vi "LDA+_An_Analysis_mode.vi"(6 "Second Graph":T2={"Plot 1"=1, "Plot 2"=2, "Save graph"=0, "Plot Type"=enum."Voltage trace"} {"Save graph" items=["Do not save plot", "Save plot"]; "Plot 2" items=["Nothing", "Prop 2 (U)"]; "Plot 1" items=["Nothing", "Prop 2 (U)"]}, 9 "First Graph":T2={"Plot 1"=1, "Plot 2"=2, "Save graph"=0, "Plot Type"=enum."Voltage trace"} {"Save graph" items=["Do not save plot", "Save plot"]; "Plot 2" items=["Nothing", "Prop 2 (U)"]; "Plot 1" items=["Nothing", "Prop 2 (U)"]}) -> (0 "Second Graph out":T2={"Plot 1"=1, "Plot 2"=2, "Save graph"=0, "Plot Type"=enum."Voltage trace"} {"Save graph" items=["Do not save plot", "Save plot"]; "Plot 2" items=["Nothing", "Prop 2 (U)"]; "Plot 1" items=["Nothing", "Prop 2 (U)"]}, 3 "First Graph out":T2={"Plot 1"=1, "Plot 2"=2, "Save graph"=0, "Plot Type"=enum."Voltage trace"} {"Save graph" items=["Do not save plot", "Save plot"]; "Plot 2" items=["Nothing", "Prop 2 (U)"]; "Plot 1" items=["Nothing", "Prop 2 (U)"]})   [LabVIEW 2010]
uses:
  Controls/Graph_Type.ctl
  Globals/Meas_global.vi
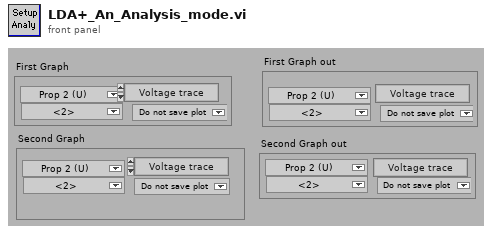
[diagram p1: front panel]
types:
  T1 = typedef "Graph_Type.ctl" = enum16{"Show no graph", "Voltage trace", "Velocity trace", "Vel histogram", "Spectrum", "f.E(f) v Log f", "Auto-Corr"}
  T2 = cluster{"Plot 1":u16, "Plot 2":u16, "Save graph":u16, "Plot Type":T1}
  T3 = typedef "Analysis_info_cluster.ctl" = cluster{"Colour":u32, "Inst type":T4, "Inst name":string, "Symbol":string, "Code name":string, "Extra Info":string, "Inst Array":T5, "Index":i32, "Voltage Index":i32, "Extra Titles":string[], "Extra Values":string[]}
  T4 = typedef "Inst_type.ctl" = enum16{"Propeller anemometer", "Raw voltage", "Pressure Transducer", "Pitot-static tube", "Preston tube", "Hot wire", "Cross wire 1", "Cross wire 2", "Generic Linear", "Generic Polynomial", "Generic BackPoly", "Fast FID", "Thermocouple", "Cold wire", "Pulsed Wire", "LDA Vel", "LDA Tran time", "LDA Arr time"}
  T5 = typedef "Instrument_Array.ctl" = enum16{"PWA", "LDA", "Analogue"}
  T6 = enum16{"Show no graph", "Voltage trace", "Velocity trace", " Vel histogram", "Spectrum", "f.E(f) v Log f", "Auto-Corr"}
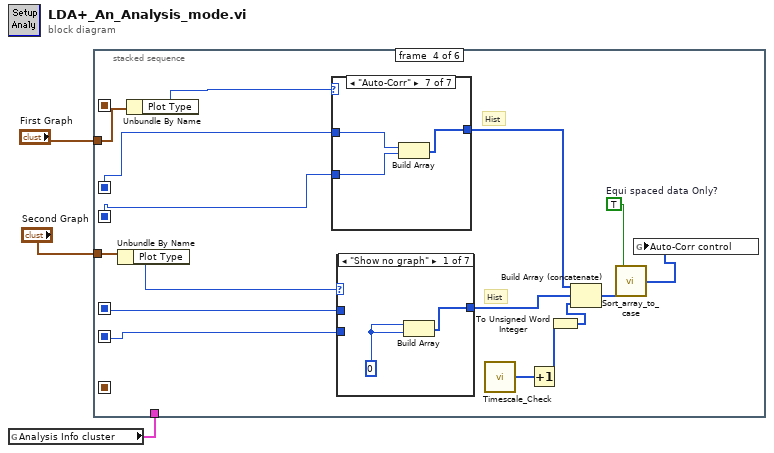
[diagram p0: block diagram]
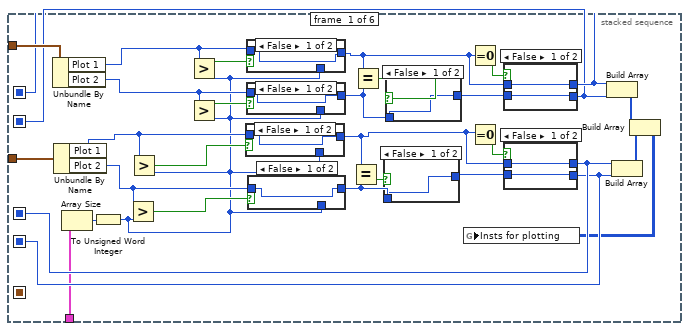
[diagram p2: hidden frame]
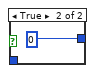
[diagram p5: hidden frame]
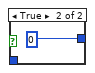
[diagram p10: hidden frame]
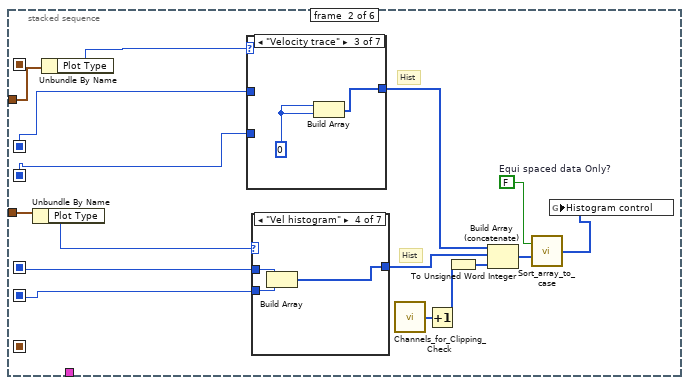
[diagram p11: hidden frame]
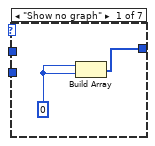
[diagram p12: hidden frame]
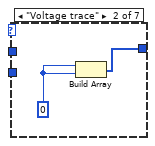
[diagram p13: hidden frame]
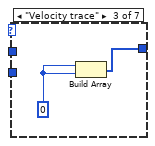
[diagram p14: hidden frame]
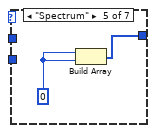
[diagram p15: hidden frame]
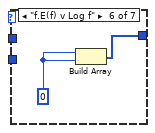
[diagram p16: hidden frame]
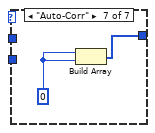
[diagram p17: hidden frame]
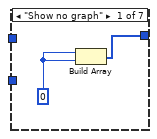
[diagram p18: hidden frame]
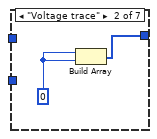
[diagram p19: hidden frame]
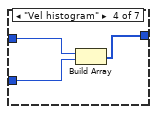
[diagram p20: hidden frame]
diagram:
  n1 = global read "Meas_global.vi" "Analysis Info cluster"() -> (w1:T3[])
  n2 = stacked-sequence {
    seq-local: [w15 _ _ _ _ _] -> [_ w64 w107 w155 w201 _]
    seq-local: [w14 _ _ _ _ _] -> [_ w63 w106 w154 w200 _]
    seq-local: [w10 _ _ _ _ _] -> [_ w66 w109 w157 w195 _]
    seq-local: [w9 _ _ _ _ _] -> [_ w65 w108 w156 w194 _]
    seq-local: [_ _ _ _ w191 _] -> [_ _ _ _ _ w229]
    seq-local: [_ _ _ _ w192 _] -> [_ _ _ _ _ w225]
    tunnel: "First Graph" -> [w24 w62 w105 w153 w204 _]
    tunnel: "Second Graph" -> [w23 w61 w104 w152 w198 _]
    tunnel: w1 -> [w4 _ _ _ _ _]
    frame #0 {
      n3 = Unbundle By Name(w24) -> ("Plot 1"=w22:u16, "Plot 2"=w21:u16)
      n4 = Unbundle By Name(w23) -> ("Plot 1"=w20:u16, "Plot 2"=w19:u16)
      n5 = Array Size(array=w4) -> (size(s)=w33:i32)
      n6 = To Unsigned Word Integer(number=w33) -> (unsigned 16bit integer=w5:u16)
      n7 = Greater?(x=w19, y=w5) -> (0:w29:bool)
      n8 = Greater?(x=w20, y=w5) -> (0:w28:bool)
      n9 = Greater?(x=w22, y=w5) -> (0:w26:bool)
      n10 = Greater?(x=w21, y=w5) -> (0:w27:bool)
      n11 = case shown="False" w28 {
        tunnel: [w48 w49] -> w12
        tunnel: w20 -> [w48 _]
        tunnel: w5 -> [_ w49]
        frame False {
        }
        frame True {
        }
      }
      n12 = case shown="False" w26 {
        tunnel: [w44 w45] -> w17
        tunnel: w22 -> [w44 _]
        tunnel: w5 -> [_ w45]
        frame False {
        }
        frame True {
        }
      }
      n13 = case shown="False" w27 {
        tunnel: [w46 w47] -> w30
        tunnel: w21 -> [w46 _]
        tunnel: w5 -> [_ w47]
        frame False {
        }
        frame True {
        }
      }
      n14 = case shown="False" w29 {
        tunnel: [w50 w51] -> w32
        tunnel: w19 -> [w50 _]
        tunnel: w5 -> [_ w51]
        frame False {
        }
        frame True {
        }
      }
      n15 = Equal?(x=w12, y=w32) -> (x = y?=w31:bool)
      n16 = Equal?(x=w17, y=w30) -> (x = y?=w25:bool)
      n17 = case shown="False" w31 {
        tunnel: [w52 u16 0] -> w11
        tunnel: w32 -> [w52 _]
        frame False {
        }
        frame True {
        }
      }
      n18 = case shown="False" w25 {
        tunnel: [w42 u16 0] -> w16
        tunnel: w30 -> [w42 _]
        frame False {
        }
        frame True {
        }
      }
      n19 = Equal To 0?(x=w17) -> (x = 0?=w18:bool)
      n20 = Equal To 0?(x=w12) -> (x = 0?=w13:bool)
      n21 = case shown="False" w18 {
        tunnel: [w38 w41] -> w14
        tunnel: w17 -> [w39 w41]
        tunnel: [w39 w40] -> w15
        tunnel: w16 -> [w38 w40]
        frame False {
        }
        frame True {
        }
      }
      n22 = case shown="False" w13 {
        tunnel: [w34 w37] -> w9
        tunnel: w12 -> [w35 w37]
        tunnel: [w35 w36] -> w10
        tunnel: w11 -> [w34 w36]
        frame False {
        }
        frame True {
        }
      }
      n23 = Build Array(w15, w14) -> (w8:u16[])
      n24 = Build Array(w10, w9) -> (w7:u16[])
      n25 = Build Array(w8, w7) -> (w6:u16[][])
      n26 = global write "Meas_global.vi" "Insts for plotting"(w6) -> ()
    }
    frame #1 {
      w54 = FALSE  # Equi spaced data Only?
      # "Hist"
      # "Hist"
      n27 = Unbundle By Name(w61) -> ("Plot Type"=w59:T1)
      n28 = Unbundle By Name(w62) -> ("Plot Type"=w60:T1)
      n29 = case shown="\"Velocity trace\"" w60 {
        tunnel: w64 -> [_ _ _ w92 _ _ _]
        tunnel: w63 -> [_ _ _ w91 _ _ _]
        tunnel: [w85 w87 w89 w93 w94 w96 w98] -> w69
        frame "Show no graph" {
          w86 = u16 0
          n30 = Build Array(w86, w86) -> (w85:u16[])
        }
        frame "Voltage trace" {
          w88 = u16 0
          n31 = Build Array(w88, w88) -> (w87:u16[])
        }
        frame "Velocity trace" {
          w90 = u16 0
          n32 = Build Array(w90, w90) -> (w89:u16[])
        }
        frame "Vel histogram" {
          n33 = Build Array(w92, w91) -> (w93:u16[])
        }
        frame "Spectrum" {
          w95 = u16 0
          n34 = Build Array(w95, w95) -> (w94:u16[])
        }
        frame "f.E(f) v Log f" {
          w97 = u16 0
          n35 = Build Array(w97, w97) -> (w96:u16[])
        }
        frame "Auto-Corr" {
          w99 = u16 0
          n36 = Build Array(w99, w99) -> (w98:u16[])
        }
      }
      n37 = case shown="\"Vel histogram\"" w59 {
        tunnel: w66 -> [_ _ _ w78 _ _ _]
        tunnel: w65 -> [_ _ _ w77 _ _ _]
        tunnel: [w70 w72 w74 w76 w79 w81 w83] -> w68
        frame "Show no graph" {
          w71 = u16 0
          n38 = Build Array(w71, w71) -> (w70:u16[])
        }
        frame "Voltage trace" {
          w73 = u16 0
          n39 = Build Array(w73, w73) -> (w72:u16[])
        }
        frame "Velocity trace" {
          w75 = u16 0
          n40 = Build Array(w75, w75) -> (w74:u16[])
        }
        frame "Vel histogram" {
          n41 = Build Array(w78, w77) -> (w76:u16[])
        }
        frame "Spectrum" {
          w80 = u16 0
          n42 = Build Array(w80, w80) -> (w79:u16[])
        }
        frame "f.E(f) v Log f" {
          w82 = u16 0
          n43 = Build Array(w82, w82) -> (w81:u16[])
        }
        frame "Auto-Corr" {
          w84 = u16 0
          n44 = Build Array(w84, w84) -> (w83:u16[])
        }
      }
      n45 = call "Channels_for_Clipping_Check.vi"() -> ("Channel Indicies"=w57:i32[])
      n46 = Increment(x=w57) -> (x+1=w55:i32[])
      n47 = To Unsigned Word Integer(number=w55) -> (unsigned 16bit integer=w56:u16[])
      n48 = Build Array (concatenate)(w69, w68, w56) -> (w67:u16[])
      n49 = call "Sort_array_to_case.vi"("Array to sort"=w67, "Equi spaced data Only?"=w54) -> ("Sorted Array"=w58:i32[])
      n50 = global write "Meas_global.vi" "Histogram control"(w58) -> ()
    }
    frame #2 {
      w100 = TRUE  # Equi spaced data Only?
      # "Hist"
      # "Hist"
      n51 = Unbundle By Name(w104) -> ("Plot Type"=w102:T1)
      n52 = Unbundle By Name(w105) -> ("Plot Type"=w103:T1)
      n53 = case shown="\"Show no graph\"" w103 {
        tunnel: w107 -> [_ _ _ _ w138 w141 _]
        tunnel: w106 -> [_ _ _ _ w137 w140 _]
        tunnel: [w129 w131 w133 w135 w139 w142 w143] -> w112
        frame "Show no graph" {
          w130 = u16 0
          n54 = Build Array(w130, w130) -> (w129:u16[])
        }
        frame "Voltage trace" {
          w132 = u16 0
          n55 = Build Array(w132, w132) -> (w131:u16[])
        }
        frame "Velocity trace" {
          w134 = u16 0
          n56 = Build Array(w134, w134) -> (w133:u16[])
        }
        frame "Vel histogram" {
          w136 = u16 0
          n57 = Build Array(w136, w136) -> (w135:u16[])
        }
        frame "Spectrum" {
          n58 = Build Array(w138, w137) -> (w139:u16[])
        }
        frame "f.E(f) v Log f" {
          n59 = Build Array(w141, w140) -> (w142:u16[])
        }
        frame "Auto-Corr" {
          w144 = u16 0
          n60 = Build Array(w144, w144) -> (w143:u16[])
        }
      }
      n61 = case shown="\"Show no graph\"" w102 {
        tunnel: w109 -> [_ _ _ _ w123 w126 _]
        tunnel: w108 -> [_ _ _ _ w122 w125 _]
        tunnel: [w113 w115 w117 w119 w121 w124 w127] -> w111
        frame "Show no graph" {
          w114 = u16 0
          n62 = Build Array(w114, w114) -> (w113:u16[])
        }
        frame "Voltage trace" {
          w116 = u16 0
          n63 = Build Array(w116, w116) -> (w115:u16[])
        }
        frame "Velocity trace" {
          w118 = u16 0
          n64 = Build Array(w118, w118) -> (w117:u16[])
        }
        frame "Vel histogram" {
          w120 = u16 0
          n65 = Build Array(w120, w120) -> (w119:u16[])
        }
        frame "Spectrum" {
          n66 = Build Array(w123, w122) -> (w121:u16[])
        }
        frame "f.E(f) v Log f" {
          n67 = Build Array(w126, w125) -> (w124:u16[])
        }
        frame "Auto-Corr" {
          w128 = u16 0
          n68 = Build Array(w128, w128) -> (w127:u16[])
        }
      }
      n69 = Build Array (concatenate)(w112, w111) -> (w110:u16[])
      n70 = call "Sort_array_to_case.vi"("Array to sort"=w110, "Equi spaced data Only?"=w100) -> ("Sorted Array"=w101:i32[])
      n71 = global write "Meas_global.vi" "Spectra control"(w101) -> ()
    }
    frame #3 {
      w148 = TRUE  # Equi spaced data Only?
      # "Hist"
      # "Hist"
      n72 = Unbundle By Name(w152) -> ("Plot Type"=w150:T1)
      n73 = Unbundle By Name(w153) -> ("Plot Type"=w151:T1)
      n74 = case shown="\"Auto-Corr\"" w151 {
        tunnel: w155 -> [_ _ _ _ _ _ w189]
        tunnel: w154 -> [_ _ _ _ _ _ w188]
        tunnel: [w176 w178 w180 w182 w184 w186 w190] -> w160
        frame "Show no graph" {
          w177 = u16 0
          n75 = Build Array(w177, w177) -> (w176:u16[])
        }
        frame "Voltage trace" {
          w179 = u16 0
          n76 = Build Array(w179, w179) -> (w178:u16[])
        }
        frame "Velocity trace" {
          w181 = u16 0
          n77 = Build Array(w181, w181) -> (w180:u16[])
        }
        frame "Vel histogram" {
          w183 = u16 0
          n78 = Build Array(w183, w183) -> (w182:u16[])
        }
        frame "Spectrum" {
          w185 = u16 0
          n79 = Build Array(w185, w185) -> (w184:u16[])
        }
        frame "f.E(f) v Log f" {
          w187 = u16 0
          n80 = Build Array(w187, w187) -> (w186:u16[])
        }
        frame "Auto-Corr" {
          n81 = Build Array(w189, w188) -> (w190:u16[])
        }
      }
      n82 = case shown="\"Show no graph\"" w150 {
        tunnel: w157 -> [_ _ _ _ _ _ w175]
        tunnel: w156 -> [_ _ _ _ _ _ w174]
        tunnel: [w161 w163 w165 w167 w169 w171 w173] -> w159
        frame "Show no graph" {
          w162 = u16 0
          n83 = Build Array(w162, w162) -> (w161:u16[])
        }
        frame "Voltage trace" {
          w164 = u16 0
          n84 = Build Array(w164, w164) -> (w163:u16[])
        }
        frame "Velocity trace" {
          w166 = u16 0
          n85 = Build Array(w166, w166) -> (w165:u16[])
        }
        frame "Vel histogram" {
          w168 = u16 0
          n86 = Build Array(w168, w168) -> (w167:u16[])
        }
        frame "Spectrum" {
          w170 = u16 0
          n87 = Build Array(w170, w170) -> (w169:u16[])
        }
        frame "f.E(f) v Log f" {
          w172 = u16 0
          n88 = Build Array(w172, w172) -> (w171:u16[])
        }
        frame "Auto-Corr" {
          n89 = Build Array(w175, w174) -> (w173:u16[])
        }
      }
      n90 = call "Timescale_Check.vi"() -> ("Channel Indicies"=w146:i32[])
      n91 = Increment(x=w146) -> (x+1=w147:i32[])
      n92 = To Unsigned Word Integer(number=w147) -> (unsigned 16bit integer=w145:u16[])
      n93 = Build Array (concatenate)(w160, w159, w145) -> (w158:u16[])
      n94 = call "Sort_array_to_case.vi"("Array to sort"=w158, "Equi spaced data Only?"=w148) -> ("Sorted Array"=w149:i32[])
      n95 = global write "Meas_global.vi" "Auto-Corr control"(w149) -> ()
    }
    frame #4 {
      n96 = Equal To 0?(x=w194) -> (x = 0?=w197:bool)
      n97 = Equal To 0?(x=w195) -> (x = 0?=w196:bool)
      n98 = Equal To 0?(x=w200) -> (x = 0?=w202:bool)
      n99 = Equal To 0?(x=w201) -> (x = 0?=w203:bool)
      n100 = And(x=w196, y=w197) -> (x .and. y?=w193:bool)
      n101 = And(x=w203, y=w202) -> (x .and. y?=w199:bool)
      n102 = case shown="False" w193 {
        tunnel: [w208 w213] -> w192
        tunnel: w194 -> [w207 w212]
        tunnel: w195 -> [w206 w211]
        tunnel: w198 -> [w205 w210]
        frame False {
          n103 = Bundle By Name(cluster=w205, "Plot 1"=w206, "Plot 2"=w207) -> (w208:T2)
        }
        frame True {
          n104 = Bundle By Name(cluster=w210, "Plot 1"=w211, "Plot 2"=w212, "Save graph"=0) -> (w213:T2)
        }
      }
      n105 = case shown="True" w199 {
        tunnel: [w217 w222] -> w191
        tunnel: w200 -> [w216 w221]
        tunnel: w201 -> [w215 w220]
        tunnel: w204 -> [w214 w219]
        frame False {
          n106 = Bundle By Name(cluster=w214, "Plot 1"=w215, "Plot 2"=w216) -> (w217:T2)
        }
        frame True {
          n107 = Bundle By Name(cluster=w219, "Plot 1"=w220, "Plot 2"=w221, "Save graph"=0) -> (w222:T2)
        }
      }
    }
    frame #5 {
      w224 = T6."Show no graph" ("Plot Type")
      n108 = Unbundle By Name(w225) -> ("Plot Type"=w226:T1)
      n109 = Unbundle By Name(w229) -> ("Plot Type"=w231:T1)
      n110 = Equal?(x=w231, y=w224) -> (x = y?=w230:bool)
      n111 = Equal?(x=w226, y=w224) -> (x = y?=w227:bool)
      n112 = case shown="True" w230 {
        tunnel: w229 -> [w236 w239]
        tunnel: [w236 w237] -> w228
        frame False {
        }
        frame True {
          n113 = Bundle By Name(cluster=w239, "Save graph"=u16 0) -> (w237:T2)
        }
      }
      "First Graph out" <- w228
      n114 = case shown="True" w227 {
        tunnel: w225 -> [w232 w235]
        tunnel: [w232 w233] -> w223
        frame False {
        }
        frame True {
          n115 = Bundle By Name(cluster=w235, "Save graph"=u16 0) -> (w233:T2)
        }
      }
      "Second Graph out" <- w223
    }
  }
